vi "UI网络流写入方端点全局.vi"() -> ()   [LabVIEW 2013]
panel:
  out "UI网络流写入方端点全局":refnum<k21>
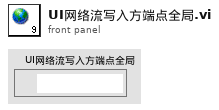
[diagram p1: front panel]
diagram:
